vi "splash_demo_v2.0.vi"() -> ()   [LabVIEW 2025]
doc: "Proof of concept/example VI for demonstration.\n\nMichael Panganiban\nSr. Hardware Test Engineer\nFresh Consulting, Inc."
uses:
  controls/home_navigation_btn.ctl
  controls/equipment_navigation_btn.ctl
  controls/settings_navigation_btn.ctl
  controls/test_plan_navigation_btn.ctl
  controls/about_button.ctl
panel:
  in  "about_button":T1
  in  "test_plan":T2
  in  "settings":T3
  in  "equipment":T4
  in  "home":T5
  in  "Tab":T6(tab)
  out "start_of_test_status":string
  in  "start_test":bool
  # "v1.0.0.1"
  # "HOME"
  # "EQUIPMENT"
  # "SETTINGS"
  # "TEST PLAN CREATION"
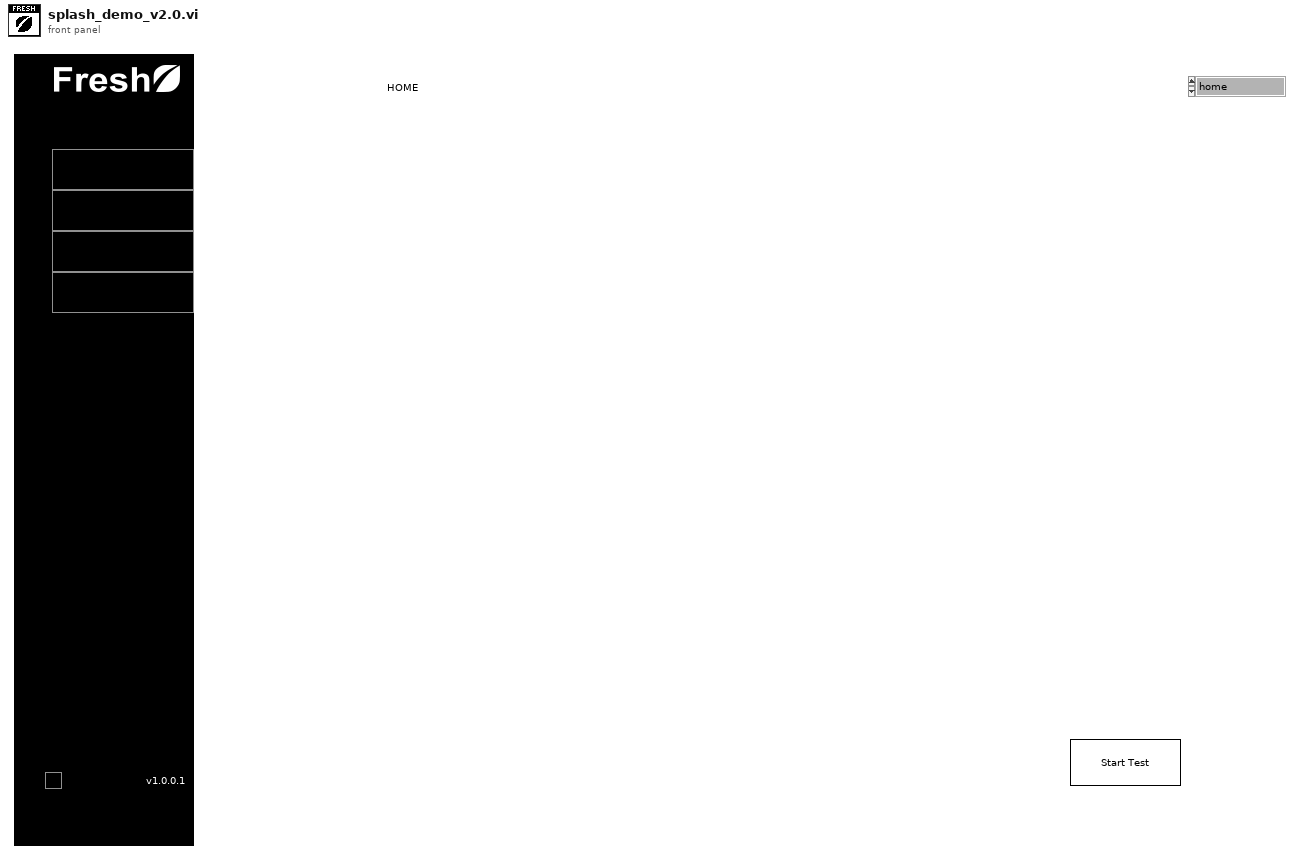
[diagram p1: front panel]
types:
  T1 = typedef "about_button.ctl" = bool
  T2 = typedef "test_plan_navigation_btn.ctl" = bool
  T3 = typedef "settings_navigation_btn.ctl" = bool
  T4 = typedef "equipment_navigation_btn.ctl" = bool
  T5 = typedef "home_navigation_btn.ctl" = bool
  T6 = enum32{"home", "equipment", "settings", "test_plan"}
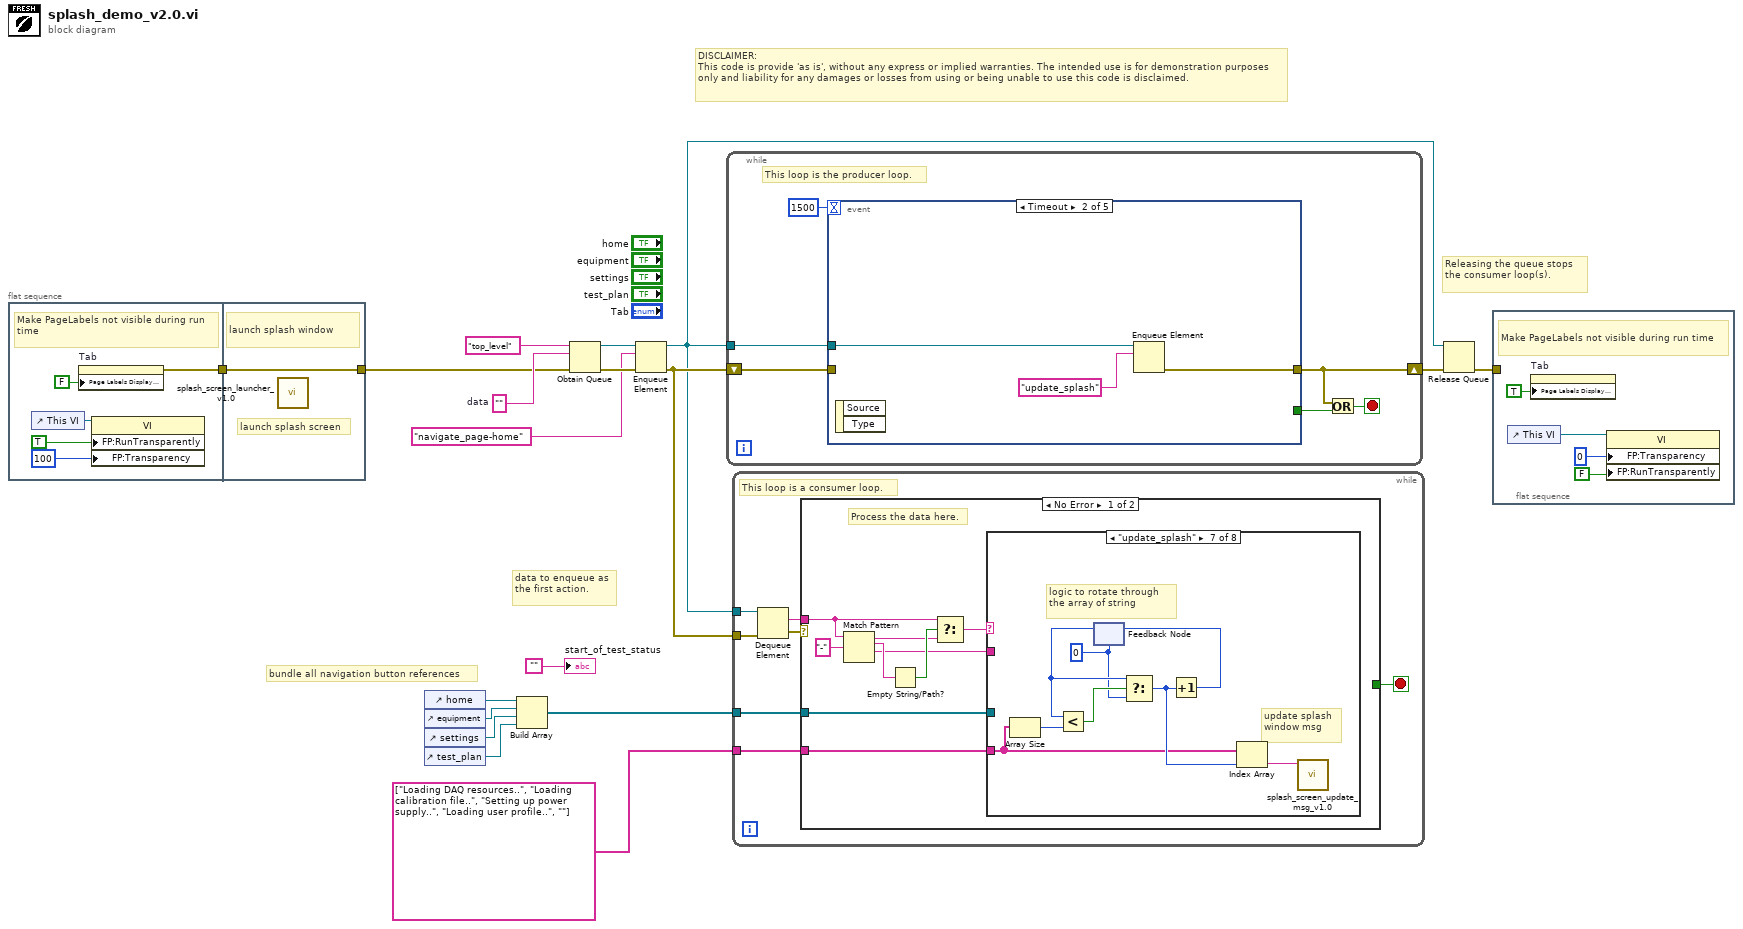
[diagram p0: block diagram]
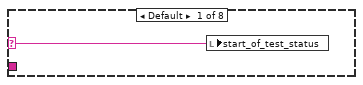
[diagram p2: hidden frame]
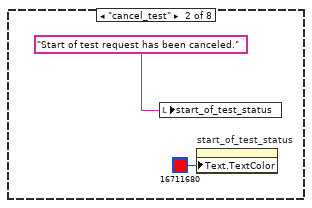
[diagram p3: hidden frame]
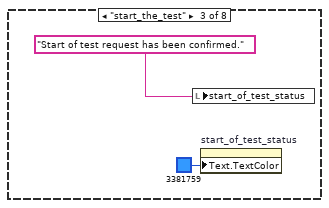
[diagram p4: hidden frame]
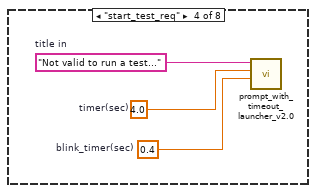
[diagram p5: hidden frame]
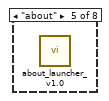
[diagram p6: hidden frame]
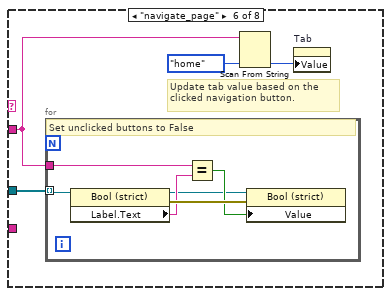
[diagram p7: hidden frame]
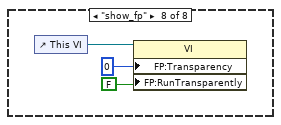
[diagram p8: hidden frame]
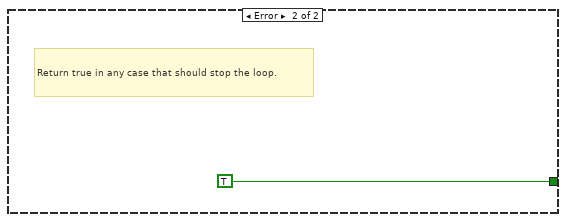
[diagram p9: hidden frame]
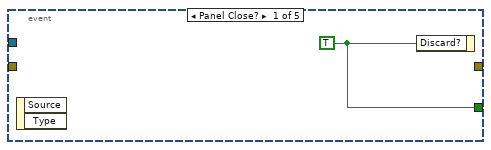
[diagram p10: hidden frame]
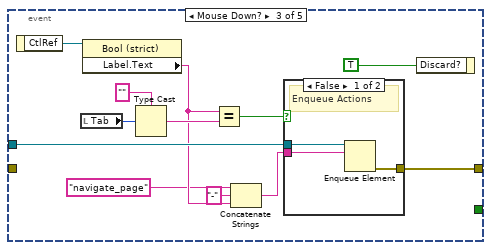
[diagram p11: hidden frame]
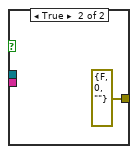
[diagram p12: hidden frame]
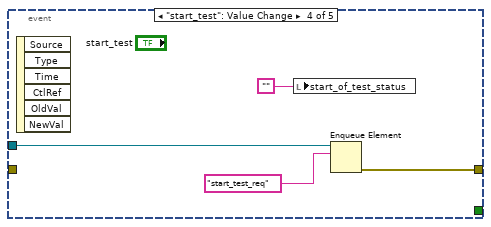
[diagram p13: hidden frame]
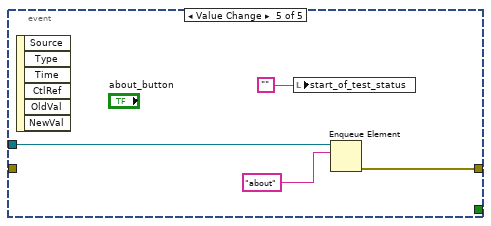
[diagram p14: hidden frame]
diagram:
  w5 = ""  # data
  # "data to enqueue as the first action."
  # "bundle all navigation button references"
  # "DISCLAIMER:\nThis code is provide 'as is', without any express or implied warranties. The intended use is for demonstration purposes only and liability for any damages or losses from using or being unable to use this code is disclaimed."
  # "Releasing the queue stops the consumer loop(s)."
  n1 = flat-sequence {
    tunnel: [w19] -> w3
    tunnel: [w24] -> w2
    tunnel: w3 -> [w24]
    frame #0 {
      # "Make PageLabels not visible during run time"
      n2 = control-ref of="This VI"() -> (w21:refnum<vi>)
      n3 = property on="Tab" class="TabCtl (strict)"("Page Labels Display Visible?"=FALSE) -> (error out=w19:errorcluster)  [unwired: 2 in, 1 out]
      n4 = property class="VI"(reference=w21, "FP:RunTransparently"=TRUE ("Front Panel Window:Run VI Transparently"), "FP:Transparency"=u8 100 ("Front Panel Window:Transparency")) -> ()  [unwired: 1 in, 2 out]
    }
    frame #1 {
      # "launch splash screen"
      # "launch splash window"
      n5 = call "splash_screen_launcher_v1.0.vi"() -> ()  [unwired: 11 in, 1 out]
    }
  }
  n6 = control-ref of="home"() -> (w10:refnum<vi>)
  n7 = control-ref of="equipment"() -> (w16:refnum<vi>)
  n8 = control-ref of="settings"() -> (w15:refnum<vi>)
  n9 = control-ref of="test_plan"() -> (w14:refnum<vi>)
  n10 = Build Array(w10, w16, w15, w14) -> (w13:refnum<vi>[])
  n11 = Obtain Queue(name (unnamed)="top_level", element data type=w5, error in (no error)=w2) -> (queue out=w12:refnum<queue>, error out=w11:errorcluster)  [unwired: 2 in, 1 out]
  n12 = Enqueue Element(queue=w12, element="navigate_page-home" ("Action"), error in (no error)=w11) -> (queue out=w8:refnum<queue>, error out=w9:errorcluster)  [unwired: 1 in, 1 out]
  n13 = while {
    shift-right: [w27] -> w18
    shift-left: w9 -> [w30]
    tunnel: w8 -> [w26]
    stop <- w28 stop-if-true
    # "This loop is the producer loop."
    n14 = event shown="[1] Timeout" {
      selector: _ -> [_ _ _ _ _]
      dyn-events: _ -> [_ _ _ _ _]
      timeout: 1500 -> [_ _ _ _ _]
      tunnel: w26 -> [_ w33 w45 w54 w58]
      tunnel: w30 -> [_ _ _ _ _]
      tunnel: [_ w32 w46 w53 w57] -> w27
      tunnel: [w31 _ _ _ _] -> w29
      event Panel Close? {
        w31 = TRUE ("Discard?")
        n15 = event-data() -> ()  [unwired: 1 in, 2 out]
        n16 = event-data("Discard?"=w31) -> ()  [unwired: 1 in, 1 out]
      }
      event Timeout {
        n17 = event-data() -> ()  [unwired: 1 in, 2 out]
        n18 = Enqueue Element(queue=w33, element="update_splash" ("Action")) -> (error out=w32:errorcluster)  [unwired: 2 in, 2 out]
      }
      event Mouse Down? {
        n19 = event-data() -> ("CtlRef"=w44:refnum<vi>)  [unwired: 1 in]
        n20 = local read "Tab"() -> (w42:T6)
        n21 = property class="Bool (strict)"(reference=w44) -> ("Label.Text"=w38:string)  [unwired: 1 in, 2 out]
        n22 = Type Cast(type="", x=w42) -> (*(type *) &x=w40:string)
        n23 = Equal?(x=w38, y=w40) -> (x = y?=w39:bool)
        n24 = Concatenate Strings("navigate_page" ("string"), "-" ("string"), w38) -> (w35:string)
        n25 = case shown="False" w39 {
          tunnel: [w49 errorcluster {"status"=FALSE, "code"=0, "source"=""} ("error out")] -> w46
          tunnel: w45 -> [w48 _]
          tunnel: w35 -> [w47 _]
          frame False {
            # "Enqueue Actions"
            n26 = Enqueue Element(queue=w48, element=w47) -> (error out=w49:errorcluster)  [unwired: 2 in, 2 out]
          }
          frame True {
          }
        }
        n27 = event-data("Discard?"=TRUE) -> ()  [unwired: 1 in, 1 out]
      }
      event "start_test": Value Change {
        n28 = event-data() -> ()  [unwired: 1 in, 6 out]
        n29 = local write "start_of_test_status"("") -> ()
        n30 = Enqueue Element(queue=w54, element="start_test_req" ("Action")) -> (error out=w53:errorcluster)  [unwired: 2 in, 2 out]
      }
      event Value Change {
        n31 = event-data() -> ()  [unwired: 1 in, 6 out]
        n32 = local write "start_of_test_status"("") -> ()
        n33 = Enqueue Element(queue=w58, element="about" ("Action")) -> (error out=w57:errorcluster)  [unwired: 2 in, 2 out]
      }
    }
    n34 = Or(x=w27, y=w29) -> (x .or. y?=w28:bool)
  }
  n35 = while {
    tunnel: w8 -> [w65]
    tunnel: w13 -> [w61]
    tunnel: w9 -> [w60]
    tunnel: string[] ["Loading DAQ resources..", "Loading calibration file..", "Setting up power supply..", "Loading user profile..", ""] -> [w59]
    stop <- w62 stop-if-true
    # "This loop is a consumer loop."
    n36 = Dequeue Element(queue=w65, error in (no error)=w60) -> (element=w63:string, error out=w64:errorcluster)  [unwired: 1 in, 2 out]
    n37 = case shown="No Error" w64 {
      tunnel: w63 -> [w70 _]
      tunnel: [_ TRUE] -> w62
      tunnel: w61 -> [w74 _]
      tunnel: w59 -> [w66 _]
      frame No Error {
        # "Process the data here."
        n38 = Match Pattern(string=w70, regular expression="-") -> (before substring=w69:string, match substring=w72:string, after substring=w67:string)  [unwired: 1 in, 1 out]
        n39 = Empty String/Path?(string/path=w72) -> (empty?=w71:bool)
        n40 = Select(t=w70, s=w71, f=w69) -> (s? t:f=w68:string)
        n41 = case shown="\"update_splash\"" w68 {
          selector: w68 -> [w75 _ _ _ _ _ _ _]
          tunnel: w74 -> [_ _ _ _ _ w84 _ _]
          tunnel: w67 -> [_ _ _ _ _ w83 _ _]
          tunnel: w66 -> [_ _ _ _ _ _ w93 _]
          frame Default {
            n42 = local write "start_of_test_status"(w75) -> ()
          }
          frame "cancel_test" {
            n43 = local write "start_of_test_status"("Start of test request has been canceled.") -> ()
            n44 = property on="start_of_test_status" class="Str"("Text.TextColor"=u32 16711680 ("Text.Text Colors:Text Color")) -> ()  [unwired: 2 in, 2 out]
          }
          frame "start_the_test" {
            n45 = local write "start_of_test_status"("Start of test request has been confirmed.") -> ()
            n46 = property on="start_of_test_status" class="Str"("Text.TextColor"=u32 3381759 ("Text.Text Colors:Text Color")) -> ()  [unwired: 2 in, 2 out]
          }
          frame "start_test_req" {
            w80 = 0.4  # blink_timer(sec)
            w81 = 4.0  # timer(sec)
            w82 = "Not valid to run a test..."  # title in
            n47 = call "prompt_with_timeout_launcher_v2.0.vi"("blink_timer(sec)"=w80, "timer(sec)"=w81, "message in"=w82) -> ()  [unwired: 8 in, 1 out]
          }
          frame "about" {
            n48 = call "about_launcher_v1.0.vi"() -> ()  [unwired: 11 in, 1 out]
          }
          frame "navigate_page" {
            # "Update tab value based on the clicked navigation button."
            n49 = for {
              tunnel: w84 -> [w92] mode=indexing
              tunnel: w83 -> [w89]
              # "Set unclicked buttons to False"
              n50 = property class="Bool (strict)"(reference=w92) -> (reference out=w87:refnum<vi>, error out=w91:errorcluster, "Label.Text"=w90:string)  [unwired: 1 in]
              n51 = Equal?(x=w89, y=w90) -> (x = y?=w88:bool)
              n52 = property class="Bool (strict)"(reference=w87, error in=w91, "Value"=w88) -> ()  [unwired: 2 out]
            }
            n53 = Scan From String(input string=w83, default 1=T6."home" ("Tab Control")) -> (output 1=w85:T6)  [unwired: 3 in, 3 out]
            n54 = property on="Tab" class="TabCtl (strict)"("Value"=w85) -> ()  [unwired: 2 in, 2 out]
          }
          frame "update_splash" {
            w94 = 0
            # "update splash window msg"
            # "logic to rotate through the array of string"
            n55 = Array Size(array=w93) -> (size(s)=w99:i32)
            n56 = feedback #1(w94) -> (w95:i32)
            n57 = Less?(x=w95, y=w99) -> (x < y?=w100:bool)
            n58 = Select(t=w95, s=w100, f=w94) -> (s? t:f=w96:i32)
            n59 = Increment(x=w96) -> (x+1=w97:i32)
            n60 = feedback-in #1(w97) -> ()
            n61 = Index Array(array=w93, index=w96) -> (element=w98:string)
            n62 = call "splash_screen_update_msg_v1.0.vi"("message in"=w98) -> ()  [unwired: 10 in, 1 out]
          }
          frame "show_fp" {
            n63 = control-ref of="This VI"() -> (w101:refnum<vi>)
            n64 = property class="VI"(reference=w101, "FP:Transparency"=u8 0 ("Front Panel Window:Transparency"), "FP:RunTransparently"=FALSE ("Front Panel Window:Run VI Transparently")) -> ()  [unwired: 1 in, 2 out]
          }
        }
      }
      frame Error {
        # "Return true in any case that should stop the loop."
      }
    }
  }
  n65 = Release Queue(queue=w8, error in (no error)=w18) -> (error out=w17:errorcluster)  [unwired: 1 in, 2 out]
  n66 = flat-sequence {
    tunnel: w17 -> [_]
    frame #0 {
      # "Make PageLabels not visible during run time"
      n67 = control-ref of="This VI"() -> (w107:refnum<vi>)
      n68 = property on="Tab" class="TabCtl (strict)"("Page Labels Display Visible?"=TRUE) -> ()  [unwired: 2 in, 2 out]
      n69 = property class="VI"(reference=w107, "FP:Transparency"=u8 0 ("Front Panel Window:Transparency"), "FP:RunTransparently"=FALSE ("Front Panel Window:Run VI Transparently")) -> ()  [unwired: 1 in, 2 out]
    }
  }
  "start_of_test_status" <- ""
